vi "If Statement structure handler.vi"(10 "function true?":bool, 11 "Auto Scripting array":T1) -> (3 "Auto Scripting array out":T1)   [LabVIEW 2013]
uses:
  Autonmous Scripting array typedef.ctl
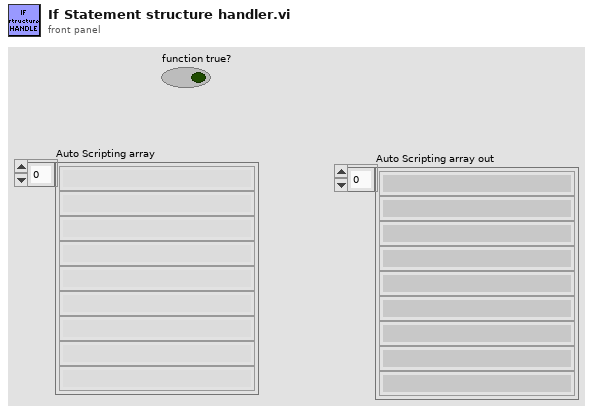
[diagram p1: front panel]
types:
  T1 = typedef "Autonmous Scripting array typedef.ctl" = string[]
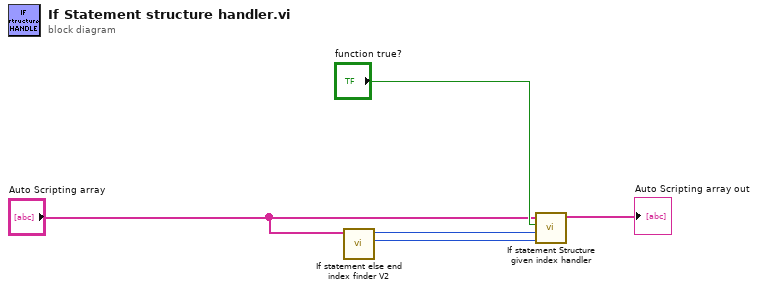
[diagram p0: block diagram]
diagram:
  n1 = call "If statement else end index finder V2.vi"("Auto Scripting array"="Auto Scripting array") -> ("end Index"=w1:i32, "else Index"=w2:i32)  [unwired: 9 in]
  n2 = call "If statement Structure given index handler.vi"("end index"=w1, "else index"=w2, "function true?"="function true?", "Auto Scripting array in"="Auto Scripting array") -> ("Auto Scripting array out"=→"Auto Scripting array out":T1)  [unwired: 7 in]
